vi "getJoystickValues.vi"(6 "Mode":enum16{"Axis", "Button"}(ring), 8 "error in (no error)":errorcluster, 9 "Axis":dbl, 10 "buttonType":enum16{"A", "B", "X", "Y", "LB", "RB"}(ring), 11 "JoystickDevRef":T1) -> (0 "error out":errorcluster, 1 "Button Pressed":bool, 2 "Value":dbl, 3 "JoystickDevRef":T1)   [LabVIEW 2016, in "External.lvlib"]
uses:
  External.lvlib
  <vilib>/Rock Robotics/WPI/Joystick/WPI_JoystickDevRef.ctl
  <vilib>/Rock Robotics/WPI/Joystick/WPI_JoystickDeviceEnum.ctl
  Index.vi
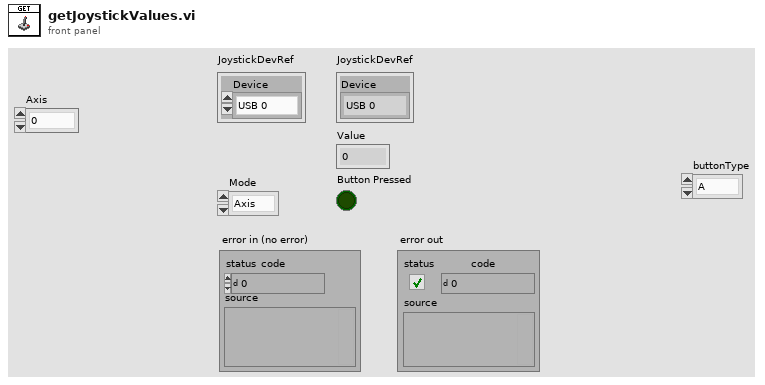
[diagram p1: front panel]
types:
  T1 = typedef "WPI_JoystickDevRef.ctl" = cluster{"Device":T2}
  T2 = typedef "WPI_JoystickDeviceEnum.ctl" = enum16{"USB 0", "USB 1", "USB 2", "USB 3", "USB 4", "USB 5"}
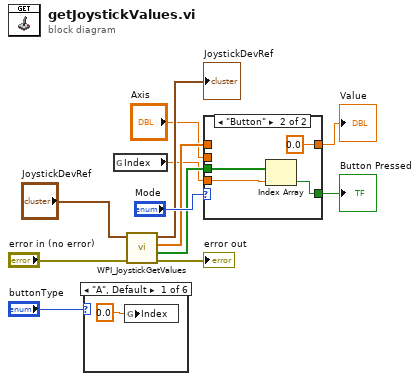
[diagram p0: block diagram]
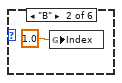
[diagram p2: hidden frame]
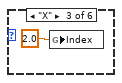
[diagram p3: hidden frame]
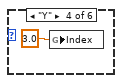
[diagram p4: hidden frame]
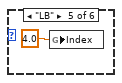
[diagram p5: hidden frame]
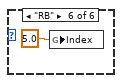
[diagram p6: hidden frame]
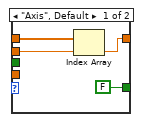
[diagram p7: hidden frame]
diagram:
  n1 = case shown="\"A\", Default" "buttonType" {
    frame "A", Default {
      n2 = global write "Index.vi" "Index"(0.0 ("Index")) -> ()
    }
    frame "B" {
      n3 = global write "Index.vi" "Index"(1.0 ("Index")) -> ()
    }
    frame "X" {
      n4 = global write "Index.vi" "Index"(2.0 ("Index")) -> ()
    }
    frame "Y" {
      n5 = global write "Index.vi" "Index"(3.0 ("Index")) -> ()
    }
    frame "LB" {
      n6 = global write "Index.vi" "Index"(4.0 ("Index")) -> ()
    }
    frame "RB" {
      n7 = global write "Index.vi" "Index"(5.0 ("Index")) -> ()
    }
  }
  n8 = global read "Index.vi" "Index"() -> (w1:dbl)
  n9 = call <vilib>:"WPI_JoystickGetValues.vi"("error in (no error)"="error in (no error)", "JoystickDevRef"="JoystickDevRef") -> ("error out"=→"error out":errorcluster, "Buttons"=w3:bool[], "Axes"=w11:dbl[], "JoystickDevRef"=→"JoystickDevRef":T1)  [unwired: 5 in, 1 out]
  n10 = case shown="\"Button\"" "Mode" {
    tunnel: w11 -> [w22 _]
    tunnel: w3 -> [_ w26]
    tunnel: "Axis" -> [w21 _]
    tunnel: [w20 0.0 ("upper limit")] -> w9
    tunnel: [FALSE w25] -> w8
    tunnel: w1 -> [_ w23]
    frame "Axis", Default {
      n11 = Index Array(array=w22, index=w21) -> (element=w20:dbl)
    }
    frame "Button" {
      n12 = Index Array(array=w26, index=w23) -> (element=w25:bool)
    }
  }
  "Value" <- w9
  "Button Pressed" <- w8
